vi "Server_FileListing.vi"(8 "error in (no error)":errorcluster, 11 "Server":path) -> (0 "error out":errorcluster, 1 "Folders":string[](array[string]), 2 "Files":string[](array[string]), 3 "File listing":string)   [LabVIEW 2020]
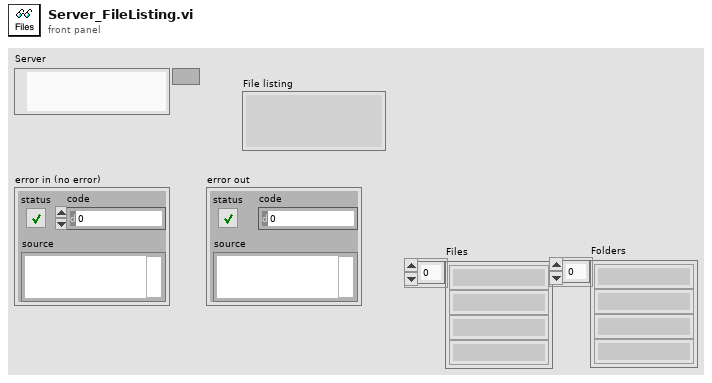
[diagram p1: front panel]
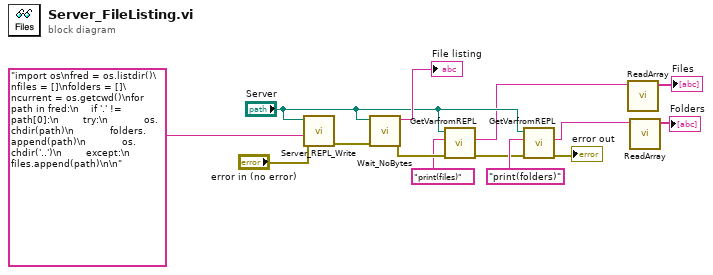
[diagram p0: block diagram]
diagram:
  n1 = call "Server_REPL_Write.vi"("error in (no error)"="error in (no error)", "Code"="import os\nfred = os.listdir()\nfiles = []\nfolders = []\ncurrent = os.getcwd()\nfor path in fred:\n    if '.' != path[0]:\n        try:\n            os.chdir(path)\n            folders.append(path)\n            os.chdir('..')\n        except:\n            files.append(path)\n\n" ("format string"), "Server"="Server") -> ("error out"=w12:errorcluster)  [unwired: 8 in]
  n2 = call "Wait_NoBytes.vi"("error in (no error)"=w12, "Server"="Server") -> ("error out"=w10:errorcluster, "String"=→"File listing":string)  [unwired: 8 in]
  n3 = call "GetVarfromREPL.vi"("error in (no error)"=w10, "Command"="print(files)", "Server"="Server") -> ("error out"=w7:errorcluster, "reply"=w4:string)  [unwired: 7 in]
  n4 = call "GetVarfromREPL.vi"("error in (no error)"=w7, "Command"="print(folders)", "Server"="Server") -> ("error out"=→"error out":errorcluster, "reply"=w2:string)  [unwired: 7 in]
  n5 = call "ReadArray.vi"("files"=w4) -> ("Files"=→"Files":string[])  [unwired: 10 in]
  n6 = call "ReadArray.vi"("files"=w2) -> ("Files"=→"Folders":string[])  [unwired: 10 in]
